vi "Read Amplitude.vi"(8 "error in (no error)":errorcluster, 11 "Composite Waveform in":refnum<class "Composite Waveform.lvclass">) -> (0 "error out":errorcluster, 2 "Amplitude":dbl, 3 "Composite Waveform out":refnum<class "Composite Waveform.lvclass">)   [LabVIEW 2020, in "Composite Waveform.lvclass"]
uses:
  Composite Waveform.lvclass
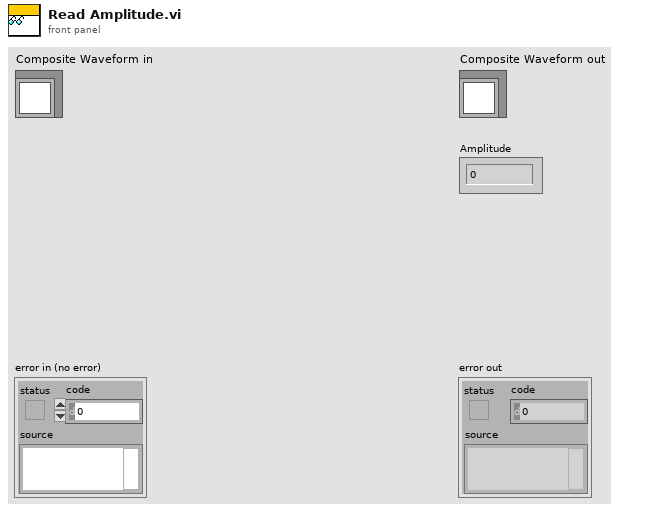
[diagram p1: front panel]
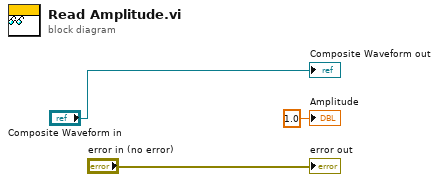
[diagram p0: block diagram]
diagram:
  "error out" <- "error in (no error)"
  "Composite Waveform out" <- "Composite Waveform in"
  "Amplitude" <- 1.0 ("Amplitude")
